vi "Tx Disable channel logic 2ch 4SPC.vi"(5 "num channels":u32, 6 "ready for output":bool, 9 "input valid":bool, 10 "data in":u32[](array[numeric])=[0, 0, 0, 0, 0, 0, 0, 0, 0, 0, 0, 0, 0, 0, 0, 0], 11 "enabled channels":u32) -> (0 "enable new data":bool, 1 "output valid":bool, 2 "data out":u32[](array[numeric]))   [LabVIEW 2025, in "niUSRP Stream Control (DMA) v1 FPGA.lvclass"]
uses:
  niUSRP Stream Control (DMA) v1 FPGA.lvclass
  niUSRP Stream Control (DMA) v1 FPGA.lvclass/niUSRP Stream Control (DMA) v1 FPGA.ctl
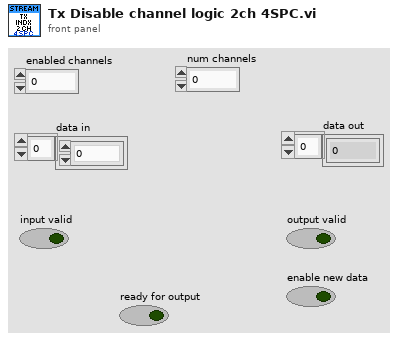
[diagram p1: front panel]
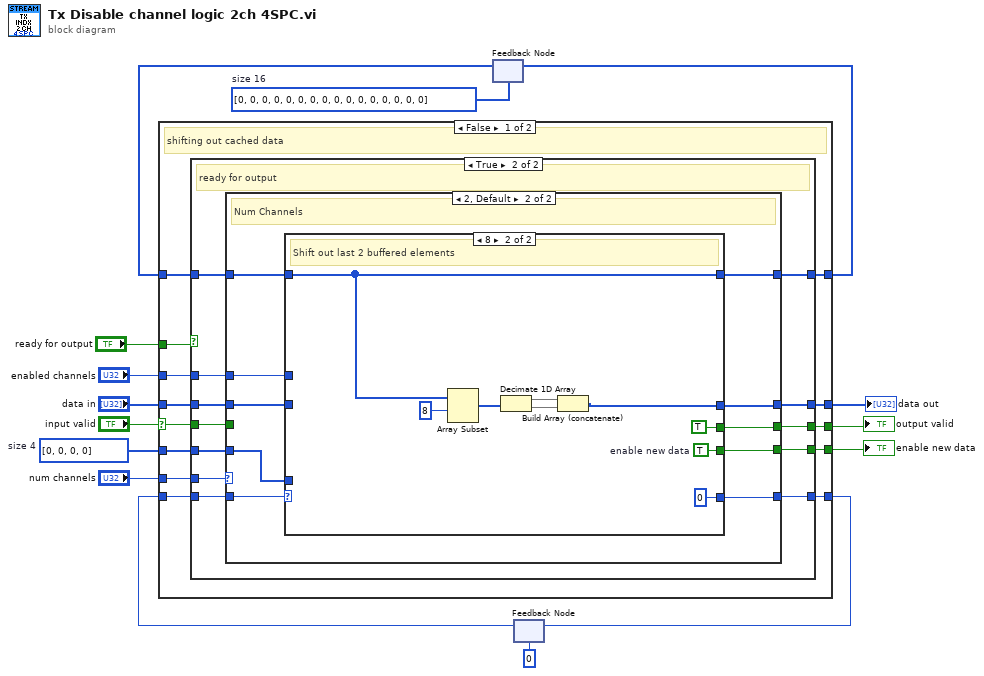
[diagram p0: block diagram]
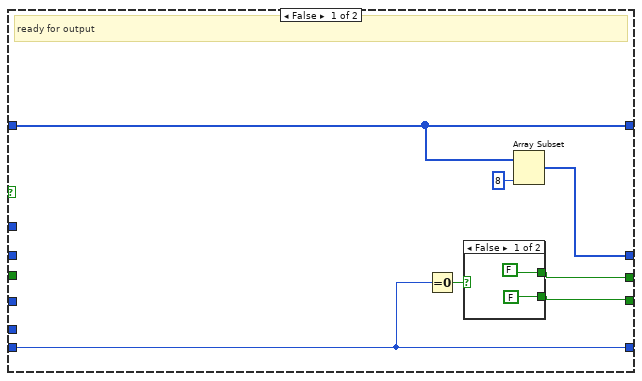
[diagram p2: hidden frame]
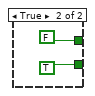
[diagram p3: hidden frame]
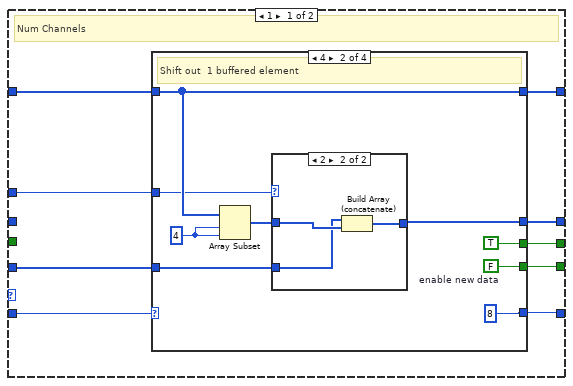
[diagram p4: hidden frame]
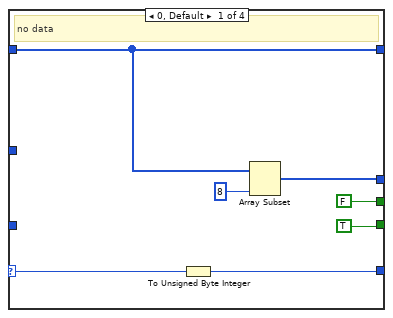
[diagram p5: hidden frame]
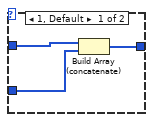
[diagram p6: hidden frame]
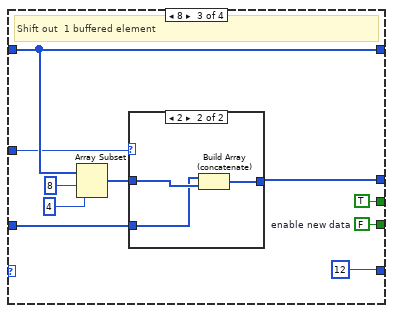
[diagram p7: hidden frame]
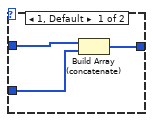
[diagram p8: hidden frame]
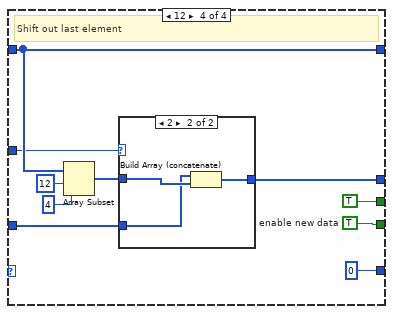
[diagram p9: hidden frame]
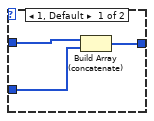
[diagram p10: hidden frame]
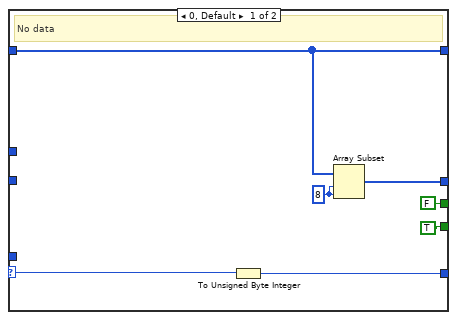
[diagram p11: hidden frame]
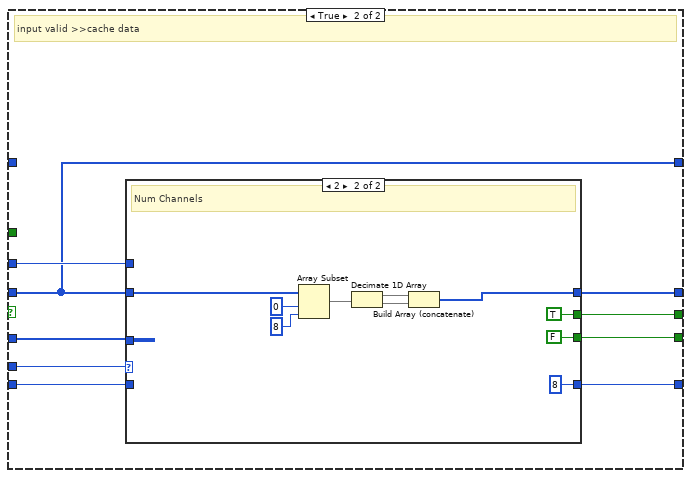
[diagram p12: hidden frame]
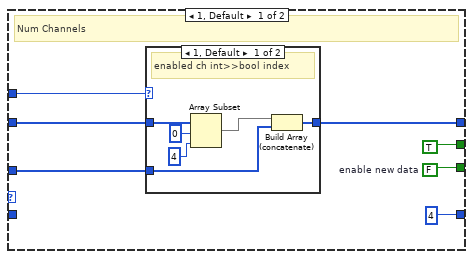
[diagram p13: hidden frame]
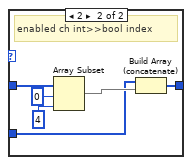
[diagram p14: hidden frame]
diagram:
  w2 = u32[] [0, 0, 0, 0]  # size 4
  w7 = u32[] [0, 0, 0, 0, 0, 0, 0, 0, 0, 0, 0, 0, 0, 0, 0, 0]  # size 16
  n1 = feedback #1(w7) -> (w6:u32[])
  n2 = feedback #2(u8 0) -> (w3:u8)
  n3 = case shown="False" "input valid" {
    selector: "input valid" -> [w18 _]
    tunnel: "num channels" -> [w28 w149]
    tunnel: [w27 w146] -> w14
    tunnel: [w26 w145] -> w13
    tunnel: "data in" -> [w25 w141]
    tunnel: "enabled channels" -> [w24 w143]
    tunnel: [w23 w144] -> w10
    tunnel: w6 -> [w22 _]
    tunnel: [w21 w141] -> w5
    tunnel: [w19 w148] -> w4
    tunnel: w3 -> [w20 w147]
    tunnel: w2 -> [w17 w142]
    tunnel: "ready for output" -> [w16 _]
    frame False {
      # "shifting out cached data"
      n4 = case shown="True" w16 {
        tunnel: w28 -> [_ w51]
        tunnel: [w33 w50] -> w27
        tunnel: [w32 w49] -> w26
        tunnel: w25 -> [_ w48]
        tunnel: w24 -> [_ w47]
        tunnel: [w29 w46] -> w23
        tunnel: w22 -> [w30 w45]
        tunnel: [w30 w44] -> w21
        tunnel: w20 -> [w34 w43]
        tunnel: [w34 w42] -> w19
        tunnel: w18 -> [_ w41]
        tunnel: w17 -> [_ w40]
        frame False {
          # "ready for output"
          n5 = Equal To 0?(x=w34) -> (x = 0?=w35:bool)
          n6 = case shown="False" w35 {
            tunnel: [FALSE TRUE] -> w32
            tunnel: [FALSE FALSE] -> w33
            frame False {
            }
            frame True {
            }
          }
          n7 = Array Subset(array=w30, length=8) -> (w29:u32[])  [unwired: 1 in]
        }
        frame True {
          # "ready for output"
          n8 = case shown="2, Default" w51 {
            tunnel: w47 -> [w58 w123]
            tunnel: w48 -> [_ w124]
            tunnel: [w54 w120] -> w49
            tunnel: [w53 w121] -> w50
            tunnel: [w52 w122] -> w46
            tunnel: w45 -> [w60 w116]
            tunnel: [w59 w117] -> w44
            tunnel: w43 -> [w56 w118]
            tunnel: [w55 w119] -> w42
            tunnel: w41 -> [_ _]
            tunnel: w40 -> [w57 w115]
            frame 1 {
              # "Num Channels"
              n9 = case shown="4" w56 {
                selector: w56 -> [w66 _ _ _]
                tunnel: [w61 u8 8 u8 12 ("length") u8 0] -> w55
                tunnel: [w62 w76 w92 w104] -> w52
                tunnel: [FALSE TRUE TRUE TRUE] -> w53
                tunnel: w60 -> [w63 w74 w90 w105]
                tunnel: [w63 w74 w90 w105] -> w59
                tunnel: [TRUE w73 w89 w106] -> w54
                tunnel: w58 -> [_ w72 w88 w103]
                tunnel: w57 -> [_ w70 w86 w101]
                frame 0, Default {
                  # "no data"
                  n10 = To Unsigned Byte Integer(number=w66) -> (unsigned 8bit integer=w61:u8)
                  n11 = Array Subset(array=w63, length=8) -> (w62:u32[])  [unwired: 1 in]
                }
                frame 4 {
                  w69 = i16 4 ("length")
                  w73 = FALSE  # enable new data
                  # "Shift out  1 buffered element"
                  n12 = Array Subset(array=w74, index=w69, length=w69) -> (w71:u32[])
                  n13 = case shown="2" w72 {
                    tunnel: [w79 w82] -> w76
                    tunnel: w71 -> [w78 w81]
                    tunnel: w70 -> [w77 w80]
                    frame 1, Default {
                      n14 = Build Array (concatenate)(w78, w77) -> (w79:u32[])
                    }
                    frame 2 {
                      n15 = Build Array (concatenate)(w80, w81) -> (w82:u32[])
                    }
                  }
                }
                frame 8 {
                  w89 = FALSE  # enable new data
                  # "Shift out  1 buffered element"
                  n16 = Array Subset(array=w90, index=i16 8 ("length"), length=i16 4) -> (w87:u32[])
                  n17 = case shown="2" w88 {
                    tunnel: [w95 w98] -> w92
                    tunnel: w87 -> [w94 w97]
                    tunnel: w86 -> [w93 w96]
                    frame 1, Default {
                      n18 = Build Array (concatenate)(w94, w93) -> (w95:u32[])
                    }
                    frame 2 {
                      n19 = Build Array (concatenate)(w96, w97) -> (w98:u32[])
                    }
                  }
                }
                frame 12 {
                  w106 = TRUE  # enable new data
                  # "Shift out last element"
                  n20 = Array Subset(array=w105, index=12, length=4) -> (w102:u32[])
                  n21 = case shown="2" w103 {
                    tunnel: [w111 w114] -> w104
                    tunnel: w102 -> [w110 w113]
                    tunnel: w101 -> [w109 w112]
                    frame 1, Default {
                      n22 = Build Array (concatenate)(w110, w109) -> (w111:u32[])
                    }
                    frame 2 {
                      n23 = Build Array (concatenate)(w112, w113) -> (w114:u32[])
                    }
                  }
                }
              }
            }
            frame 2, Default {
              # "Num Channels"
              n24 = case shown="8" w118 {
                selector: w118 -> [w130 _]
                tunnel: w124 -> [_ _]
                tunnel: [w129 u8 0] -> w119
                tunnel: [w126 w132] -> w122
                tunnel: [FALSE TRUE] -> w121
                tunnel: w116 -> [w127 w133]
                tunnel: [w127 w133] -> w117
                tunnel: [TRUE w138] -> w120
                tunnel: w123 -> [_ _]
                tunnel: w115 -> [_ _]
                frame 0, Default {
                  w125 = 8 ("length")
                  # "No data"
                  n25 = To Unsigned Byte Integer(number=w130) -> (unsigned 8bit integer=w129:u8)
                  n26 = Array Subset(array=w127, index=w125, length=w125) -> (w126:u32[])
                }
                frame 8 {
                  w138 = TRUE  # enable new data
                  # "Shift out last 2 buffered elements"
                  n27 = Array Subset(array=w133, index=i16 8 ("y")) -> (w136:u32[])  [unwired: 1 in]
                  n28 = Decimate 1D Array(w136) -> (w135:u32[], w134:u32[])
                  n29 = Build Array (concatenate)(w135, w134) -> (w132:u32[])
                }
              }
            }
          }
        }
      }
    }
    frame True {
      # "input valid >>cache data"
      n30 = case shown="2" w149 {
        tunnel: [u8 4 ("x") u8 8 ("length")] -> w148
        tunnel: w147 -> [_ _]
        tunnel: w141 -> [w152 w170]
        tunnel: [TRUE TRUE] -> w146
        tunnel: [w155 FALSE ("enable new data")] -> w145
        tunnel: [w150 w169] -> w144
        tunnel: w143 -> [w153 _]
        tunnel: w142 -> [w151 _]
        frame 1, Default {
          w155 = FALSE  # enable new data
          # "Num Channels"
          n31 = case shown="1, Default" w153 {
            tunnel: [w160 w167] -> w150
            tunnel: w152 -> [w162 w168]
            tunnel: w151 -> [w159 w165]
            frame 1, Default {
              # "enabled ch int>>bool index"
              n32 = Array Subset(array=w162, index=i16 0, length=4) -> (w161:u32[])
              n33 = Build Array (concatenate)(w161, w159) -> (w160:u32[])
            }
            frame 2 {
              # "enabled ch int>>bool index"
              n34 = Array Subset(array=w168, index=i16 0, length=4) -> (w166:u32[])
              n35 = Build Array (concatenate)(w165, w166) -> (w167:u32[])
            }
          }
        }
        frame 2 {
          # "Num Channels"
          n36 = Array Subset(array=w170, index=i16 0 ("y"), length=i16 8 ("y")) -> (w173:u32[])
          n37 = Decimate 1D Array(w173) -> (w172:u32[], w171:u32[])
          n38 = Build Array (concatenate)(w172, w171) -> (w169:u32[])
        }
      }
    }
  }
  "output valid" <- w14
  "enable new data" <- w13
  "data out" <- w10
  n39 = feedback-in #1(w5) -> ()
  n40 = feedback-in #2(w4) -> ()
